vi "Update.vi"(8 "error in (no error)":errorcluster, 11 "Game in":refnum<class "Game.lvclass">) -> (0 "error out":errorcluster, 3 "Game out":refnum<class "Game.lvclass">)   [LabVIEW 2019, in "RT_Game.lvlib" / "Game.lvclass"]
uses:
  Game.lvclass
  Game.lvclass/Game.ctl
  <vilib>/Utility/error.llb/Error Cluster From Error Code.vi
  <vilib>/rvi/errors/niLvFpgaAdjustHostInterfaceError.vi
  <vilib>/rvi/interface/nirviReadWriteControl/nirviReadWriteControl.xnode
  FPGA_Interface.ctl
  FPGA Bitfiles/myriogameconsole_FPGATarget_Main_ntsPRcBZGxk.lvbitx
  RT_Sprite/RT_Sprite.lvclass
  NiFpgaLv.dll
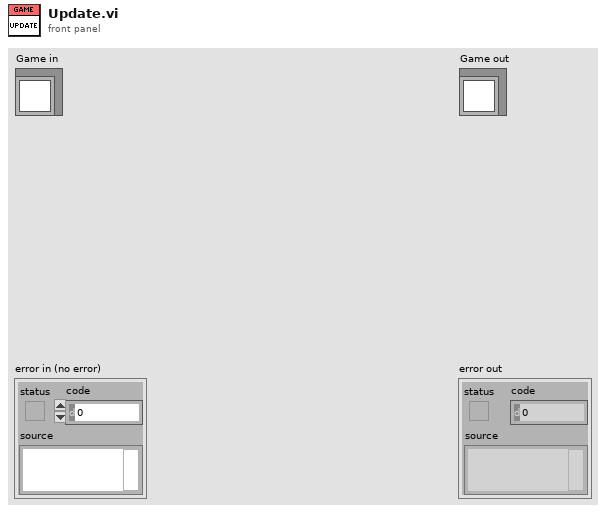
[diagram p1: front panel]
types:
  T1 = typedef "FPGA_Interface.ctl" = refnum<k20>
  T2 = typedef "RT_Game.lvlib/Game.lvclass/SpritesCluster.ctl" = cluster{"Sprite1":refnum<class "RT_Sprite.lvclass">, "Sprite2":refnum<class "RT_Sprite.lvclass">, "Sprite3":refnum<class "RT_Sprite.lvclass">}
  T3 = cluster{"[0]":refnum<class "RT_Sprite.lvclass">, "[1]":refnum<class "RT_Sprite.lvclass">, "[2]":refnum<class "RT_Sprite.lvclass">}
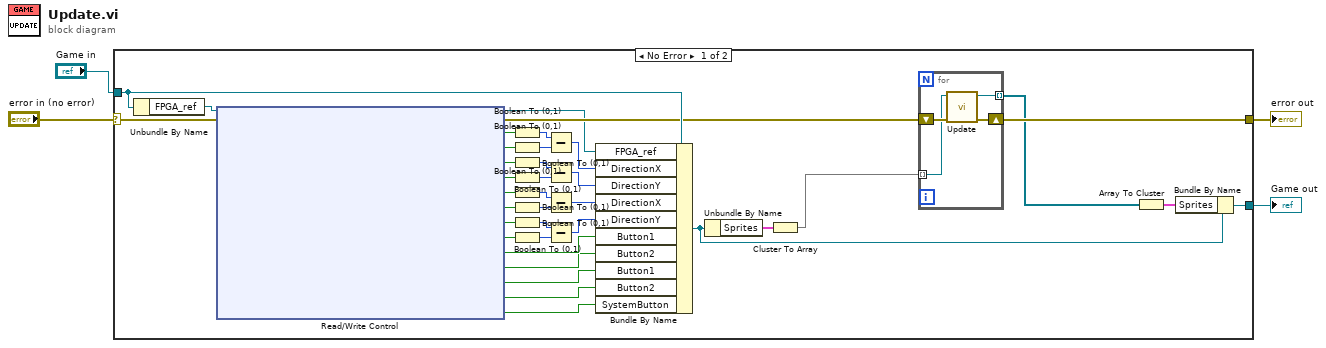
[diagram p0: block diagram]
diagram:
  n1 = case shown="No Error" "error in (no error)" {
    selector: "error in (no error)" -> [w41 w47]
    tunnel: [w9 w47] -> w3
    tunnel: [w7 w46] -> w1
    tunnel: "Game in" -> [w40 w46]
    frame No Error {
      n2 = Unbundle By Name(w40) -> ("FPGA_ref"=w12:T1)
      n3 = xnode "Read/Write Control"("FPGA VI Reference In"=w12, "error in"=w41) -> ("FPGA VI Reference Out"=w30:T1, "error out"=w39:errorcluster, "left_right"=w38:bool, "left_left"=w37:bool, "left_down"=w26:bool, "left_up"=w25:bool, "right_right"=w32:bool, "right_left"=w31:bool, "right_down"=w22:bool, "right_up"=w21:bool, "left_1"=w18:bool, "left_2"=w17:bool, "right_1"=w16:bool, "right_2"=w15:bool, "SystemButton"=w13:bool)
      n4 = Boolean To (0,1)(Boolean=w38) -> (0, 1=w36:i16)
      n5 = Boolean To (0,1)(Boolean=w37) -> (0, 1=w35:i16)
      n6 = Boolean To (0,1)(Boolean=w26) -> (0, 1=w27:i16)
      n7 = Boolean To (0,1)(Boolean=w25) -> (0, 1=w28:i16)
      n8 = Boolean To (0,1)(Boolean=w32) -> (0, 1=w33:i16)
      n9 = Boolean To (0,1)(Boolean=w31) -> (0, 1=w34:i16)
      n10 = Boolean To (0,1)(Boolean=w22) -> (0, 1=w14:i16)
      n11 = Boolean To (0,1)(Boolean=w21) -> (0, 1=w23:i16)
      n12 = Subtract(x=w36, y=w35) -> (x-y=w29:i16)
      n13 = Subtract(x=w27, y=w28) -> (x-y=w24:i16)
      n14 = Subtract(x=w33, y=w34) -> (x-y=w20:i16)
      n15 = Subtract(x=w14, y=w23) -> (x-y=w19:i16)
      n16 = Bundle By Name(cluster=w40, "FPGA_ref"=w30, "DirectionX"=w29, "DirectionY"=w24, "DirectionX"=w20, "DirectionY"=w19, "Button1"=w18, "Button2"=w17, "Button1"=w16, "Button2"=w15, "SystemButton"=w13) -> (w11:refnum<class "Game.lvclass">)
      n17 = Unbundle By Name(w11) -> ("Sprites"=w10:T2)
      n18 = Cluster To Array(cluster=w10) -> (array=w8:refnum<class "RT_Sprite.lvclass">[])
      n19 = for {
        tunnel: w8 -> [w43] mode=indexing
        tunnel: [w42] -> w6 mode=indexing
        shift-right: [w44] -> w9
        shift-left: w39 -> [w45]
        n20 = call-dynamic "Update.vi"("error in (no error)"=w45, "GameObject in"=w43) -> ("error out"=w44:errorcluster, "GameObject out"=w42:refnum<class "RT_Sprite.lvclass">)  [unwired: 8 in]
      }
      n21 = Array To Cluster(array=w6) -> (cluster=w5:T3)
      n22 = Bundle By Name(cluster=w11, "Sprites"=w5) -> (w7:refnum<class "Game.lvclass">)
    }
    frame Error {
    }
  }
  "error out" <- w3
  "Game out" <- w1
